vi "NewTarget.vi"(0 "Target x":dbl, 5 "Target y":dbl, 7 "Current x":dbl, 9 "Current y":dbl, 11 "error in (no error)":errorcluster) -> (4 "NewTarget":bool, 15 "error out":errorcluster)   [LabVIEW 2017, in "admittanceControllerLibrary.lvlib"]
doc: "Checks to see whether this is a new reaching target.\n\nIf it is a new target, reinitialises some parameters necessary for a minimum jerk trajectory"
uses:
  admittanceControllerLibrary.lvlib
  Controls/timer control.ctl
  Controls/initial conditions control.ctl
  Controls/tf control.ctl
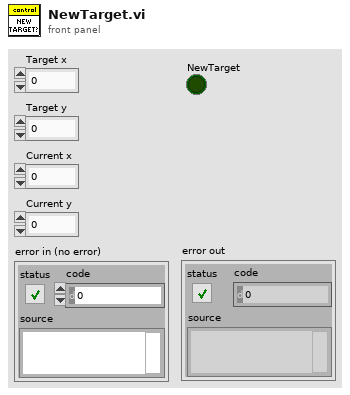
[diagram p1: front panel]
types:
  T1 = typedef "admittanceControllerLibrary.lvlib/timer control.ctl" = enum16{"get time", "set time"}
  T2 = typedef "admittanceControllerLibrary.lvlib/tf control.ctl" = enum16{"get tf", "set tf"}
  T3 = typedef "admittanceControllerLibrary.lvlib/initial conditions control.ctl" = enum16{"get", "set"}
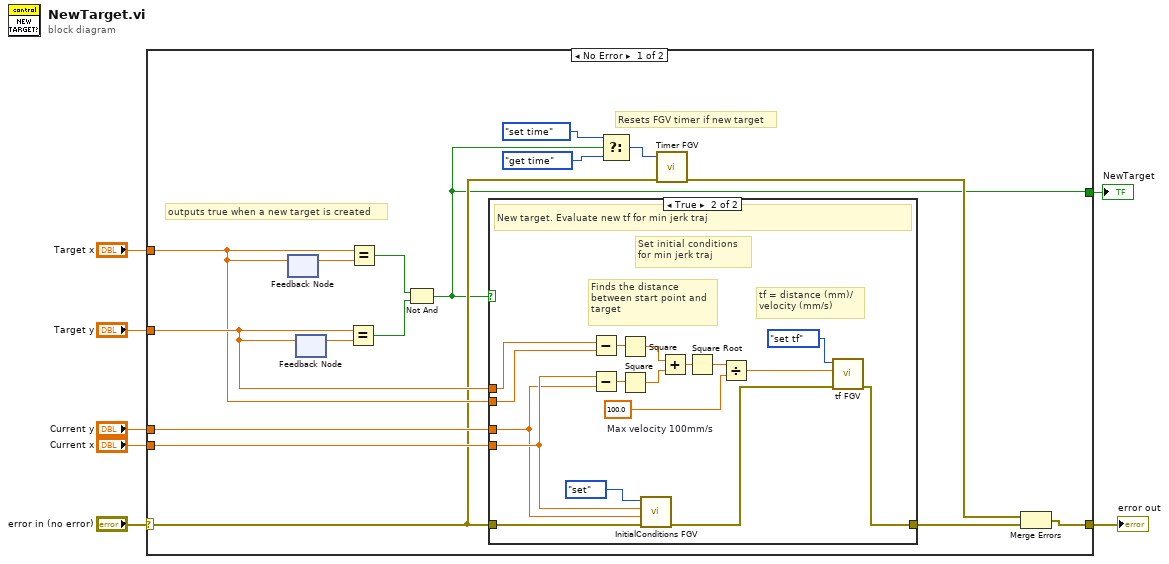
[diagram p0: block diagram]
diagram:
  n1 = case shown="No Error" "error in (no error)" {
    selector: "error in (no error)" -> [w12 w42]
    tunnel: "Target y" -> [w19 _]
    tunnel: "Target x" -> [w18 _]
    tunnel: "Current y" -> [w17 _]
    tunnel: "Current x" -> [w16 _]
    tunnel: [w11 w42] -> w2
    tunnel: [w8 _] -> w1
    frame No Error {
      # "Resets FGV timer if new target"
      # "outputs true when a new target is created"
      n2 = feedback #1() -> (w23:dbl)  [unwired: 1 in]
      n3 = feedback-in #1(w18) -> ()
      n4 = feedback #2() -> (w22:dbl)  [unwired: 1 in]
      n5 = feedback-in #2(w19) -> ()
      n6 = Equal?(x=w19, y=w22) -> (x = y?=w20:bool)
      n7 = Equal?(x=w18, y=w23) -> (x = y?=w21:bool)
      n8 = Not And(1:w20, 2:w21) -> (0:w8:bool)
      n9 = case shown="True" w8 {
        tunnel: w19 -> [_ w36]
        tunnel: w18 -> [_ w35]
        tunnel: w17 -> [_ w30]
        tunnel: w16 -> [_ w31]
        tunnel: w12 -> [w24 w27]
        tunnel: [w24 w25] -> w9
        frame False {
          # "Not a new target. Do nothing"
        }
        frame True {
          w33 = 100.0  # Max velocity 100mm/s
          # "Finds the distance\nbetween start point and\ntarget"
          # "Set initial conditions\nfor min jerk traj"
          # "tf = distance (mm)/\nvelocity (mm/s)"
          # "New target. Evaluate new tf for min jerk traj"
          n10 = Subtract(x=w36, y=w35) -> (x-y=w41:dbl)
          n11 = Subtract(x=w31, y=w30) -> (x-y=w40:dbl)
          n12 = Square(x=w41) -> (x^2=w39:dbl)
          n13 = Square(x=w40) -> (x^2=w38:dbl)
          n14 = call "InitialConditions FGV.vi"("error in (no error)"=w27, "Y0"=w30, "X0"=w31, "Enum"=initial_conditions_control."set") -> ("error out"=w26:errorcluster)  [unwired: 5 in, 2 out]
          n15 = Add(x=w39, y=w38) -> (x+y=w37:dbl)
          n16 = Square Root(x=w37) -> (sqrt(x)=w34:dbl)
          n17 = Divide(x=w34, y=w33) -> (x/y=w32:dbl)
          n18 = call "tf FGV.vi"("error in (no error)"=w26, "set tf"=w32, "Enum"=tf_control."set tf") -> ("error out"=w25:errorcluster)  [unwired: 7 in, 1 out]
        }
      }
      n19 = Select(t=timer_control."set time" ("Enum"), s=w8, f=timer_control."get time" ("Enum")) -> (s? t:f=w13:T1)
      n20 = call "Timer FGV.vi"("error in (no error)"=w12, "Enum"=w13) -> ("error out"=w10:errorcluster)  [unwired: 8 in, 1 out]
      n21 = Merge Errors(w10, w9) -> (w11:errorcluster)
    }
    frame Error {
    }
  }
  "error out" <- w2
  "NewTarget" <- w1
